vi "MT_Rel.vi"(8 "Error In":errorcluster caption="错误输入", 10 "Y轴偏移(μm)":dbl, 11 "X轴偏移(μm)":dbl) -> (0 "Error Out":errorcluster caption="错误输出")   [LabVIEW 2020]
uses:
  lib/MT/MT_API.lvlib
panel:
  out "Y轴位置(mm)":dbl
  out "X轴位置(mm)":dbl
  # "将设备移动到偏移位置\n并等待其移动完成"
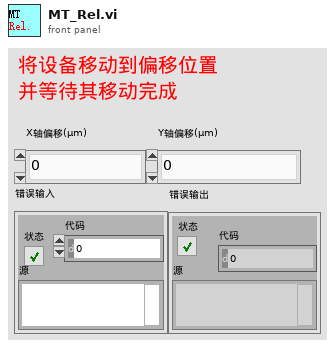
[diagram p1: front panel]
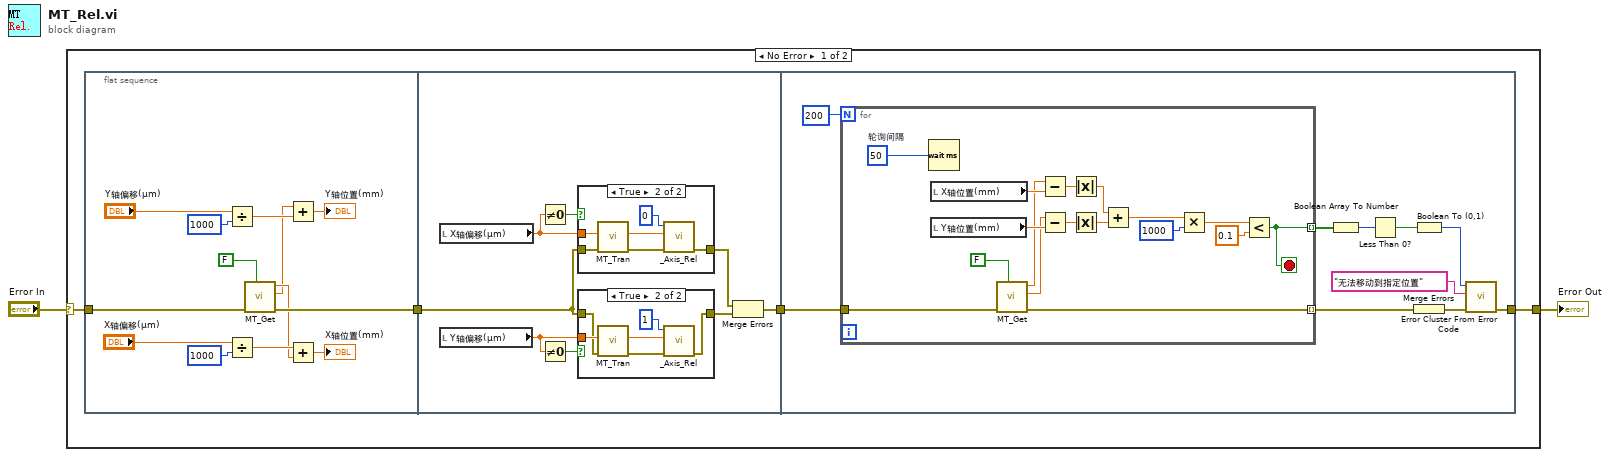
[diagram p0: block diagram]
diagram:
  n1 = case shown="No Error" "Error In" {
    selector: "Error In" -> [w6 w69]
    tunnel: [w3 w69] -> w1
    frame No Error {
      n2 = flat-sequence {
        tunnel: w6 -> [w19]
        tunnel: [w18] -> w4
        tunnel: [w22] -> w5
        tunnel: w4 -> [w23]
        tunnel: w5 -> [w43]
        tunnel: [w42] -> w3
        frame #0 {
          n3 = Divide(x="Y轴偏移(μm)", y=1000) -> (x/y=w11:dbl)
          n4 = Divide(x="X轴偏移(μm)", y=1000) -> (x/y=w12:dbl)
          n5 = call "MT_Get.vi"("手动操作(False)"=FALSE, "Error In"=w19) -> ("Error Out"=w18:errorcluster, "Y轴位置"=w7:dbl, "X轴位置"=w8:dbl)  [unwired: 5 in, 2 out]
          n6 = Add(x=w7, y=w11) -> (x+y=→"Y轴位置(mm)":dbl)
          n7 = Add(x=w12, y=w8) -> (x+y=→"X轴位置(mm)":dbl)
        }
        frame #1 {
          n8 = local read "X轴偏移(μm)"() -> (w21:dbl)
          n9 = local read "Y轴偏移(μm)"() -> (w20:dbl)
          n10 = Not Equal To 0?(x=w21) -> (x != 0?=w27:bool)
          n11 = Not Equal To 0?(x=w20) -> (x != 0?=w26:bool)
          n12 = case shown="True" w27 {
            tunnel: w21 -> [_ w40]
            tunnel: w23 -> [w35 w37]
            tunnel: [w35 w38] -> w25
            frame False {
            }
            frame True {
              n13 = call "MT_Tran.vi"("Error In"=w37, "偏移量(μm)"=w40) -> ("Error Out"=w39:errorcluster, "脉冲个数"=w41:dbl)  [unwired: 6 in, 2 out]
              n14 = call "_Axis_Rel.vi"("Error In"=w39, "相对位置"=w41, "轴序号"=0) -> ("Error Out"=w38:errorcluster)  [unwired: 8 in]
            }
          }
          n15 = case shown="True" w26 {
            tunnel: w20 -> [_ w33]
            tunnel: w23 -> [w28 w30]
            tunnel: [w28 w31] -> w24
            frame False {
            }
            frame True {
              n16 = call "MT_Tran.vi"("Error In"=w30, "偏移量(μm)"=w33) -> ("Error Out"=w32:errorcluster, "脉冲个数"=w34:dbl)  [unwired: 6 in, 2 out]
              n17 = call "_Axis_Rel.vi"("Error In"=w32, "相对位置"=w34, "轴序号"=1) -> ("Error Out"=w31:errorcluster)  [unwired: 8 in]
            }
          }
          n18 = Merge Errors(w25, w24) -> (w22:errorcluster)
        }
        frame #2 {
          n19 = for {
            N: 200 -> [_]
            tunnel: w43 -> [w68]
            tunnel: [w60] -> w51 mode=indexing
            tunnel: [w59] -> w49 mode=indexing
            stop <- w60 stop-if-true
            w58 = 50  # 轮询间隔
            n20 = Wait (ms)(milliseconds to wait=w58) -> ()  [unwired: 1 out]
            n21 = local read "X轴位置(mm)"() -> (w67:dbl)
            n22 = local read "Y轴位置(mm)"() -> (w62:dbl)
            n23 = call "MT_Get.vi"("手动操作(False)"=FALSE, "Error In"=w68) -> ("Error Out"=w59:errorcluster, "Y轴位置"=w52:dbl, "X轴位置"=w53:dbl)  [unwired: 5 in, 2 out]
            n24 = Subtract(x=w53, y=w67) -> (x-y=w65:dbl)
            n25 = Subtract(x=w52, y=w62) -> (x-y=w64:dbl)
            n26 = Absolute Value(x=w65) -> (abs(x)=w66:dbl)
            n27 = Absolute Value(x=w64) -> (abs(x)=w63:dbl)
            n28 = Add(x=w66, y=w63) -> (x+y=w56:dbl)
            n29 = Multiply(x=w56, y=1000) -> (x*y=w55:dbl)
            n30 = Less?(x=w55, y=0.1) -> (x < y?=w60:bool)
          }
          n31 = Boolean Array To Number(Boolean array=w51) -> (number=w47:u32)
          n32 = Less Than 0?(x=w47) -> (x < 0?=w46:bool)
          n33 = Boolean To (0,1)(Boolean=w46) -> (0, 1=w45:i16)
          n34 = Merge Errors(w49) -> (w48:errorcluster)
          n35 = call <vilib>:"Error Cluster From Error Code.vi"("error in (no error)"=w48, "error message (\"\")"="无法移动到指定位置", "error code (0)"=w45) -> ("error out"=w42:errorcluster)  [unwired: 6 in]
        }
      }
    }
    frame Error {
    }
  }
  "Error Out" <- w1
